vi "ma_sml_Interpolation by Zero Insert (complex input).vi"(1 "L":i32, 2 "x":cdb[](array[numeric]) format="%.2f") -> (0 "y":cdb[](array[numeric]) format="%.2f")   [LabVIEW 2020, in "NI_MAPro.lvlib"]
uses:
  NI_MAPro.lvlib
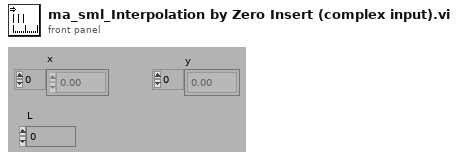
[diagram p1: front panel]
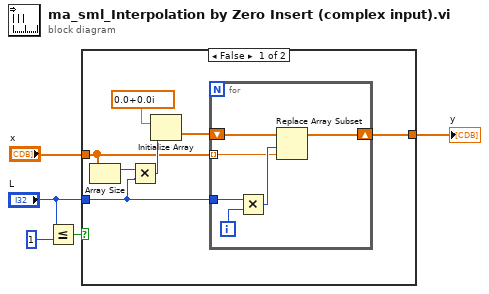
[diagram p0: block diagram]
diagram:
  n1 = Less Or Equal?(x="L", y=1) -> (x <= y?=w1:bool)
  n2 = case shown="False" w1 {
    tunnel: "x" -> [w9 w19]
    tunnel: "L" -> [w7 _]
    tunnel: [w6 w19] -> w4
    frame False {
      n3 = Array Size(array=w9) -> (size(s)=w8:i32)
      n4 = Multiply(x=w8, y=w7) -> (x*y=w11:i32)
      n5 = Initialize Array(cdb 0.0+0.0i ("Element Data"), w11) -> (w10:cdb[])
      n6 = for {
        shift-right: [w16] -> w6
        shift-left: w10 -> [w17]
        tunnel: w9 -> [w13] mode=indexing
        tunnel: w7 -> [w14]
        i -> [w18]
        n7 = Multiply(x=w14, y=w18) -> (x*y=w15:i32)
        n8 = Replace Array Subset(array=w17, new element=w13, index=w15) -> (w16:cdb[])
      }
    }
    frame True {
    }
  }
  "y" <- w4
